vi "parse_string.vi"(8 "Error In":errorcluster, 11 "Input String":string) -> (0 "Error Out":errorcluster, 2 "Displacement":dbl, 3 "Time":dbl)   [LabVIEW 2021]
doc: "Parse the serial string."
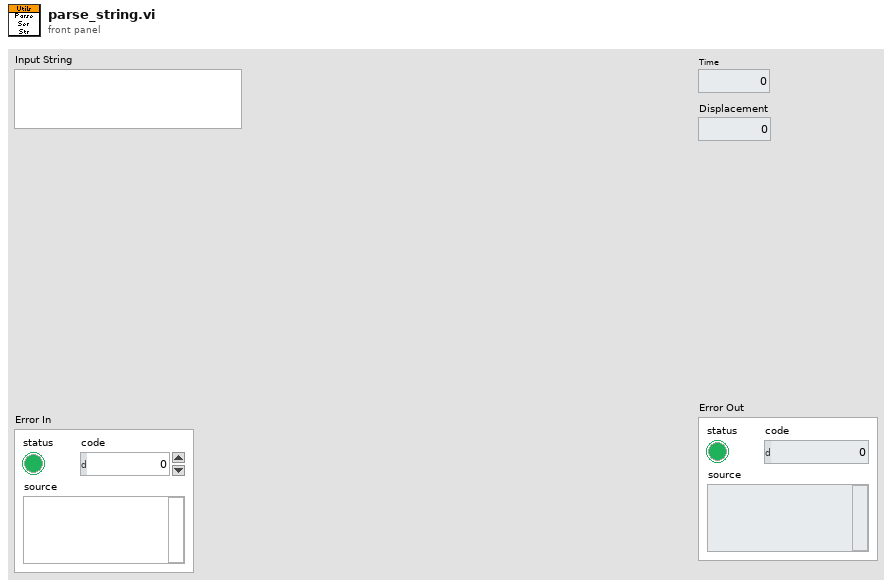
[diagram p1: front panel]
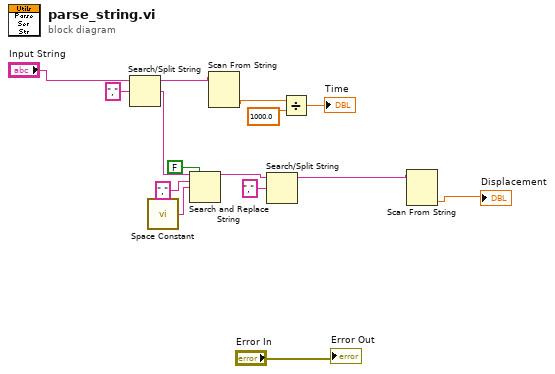
[diagram p0: block diagram]
diagram:
  n1 = Search/Split String(string="Input String", search string/char (-)=",") -> (substring before match=w2:string, match + rest of string=w6:string)  [unwired: 1 in, 1 out]
  n2 = call <vilib>:"Space Constant.vi"() -> ("String"=w9:string)
  n3 = Search and Replace String(replace all?=FALSE ("replace all? (F)"), input string=w6, search string=",", replace string=w9) -> (result string=w5:string)  [unwired: 4 in, 3 out]
  n4 = Scan From String(input string=w2) -> (output 1=w1:dbl)  [unwired: 4 in, 3 out]
  n5 = Search/Split String(string=w5, search string/char (-)=",") -> (substring before match=w3:string)  [unwired: 1 in, 2 out]
  n6 = Divide(x=w1, y=1000.0) -> (x/y=→"Time":dbl)
  n7 = Scan From String(input string=w3) -> (output 1=→"Displacement":dbl)  [unwired: 4 in, 3 out]
  "Error Out" <- "Error In"
